vi "ograniczenie pwm6.vi"(10 "button 1":bool, 11 "X axis":i32) -> (3 "y":i16)   [LabVIEW 2015]
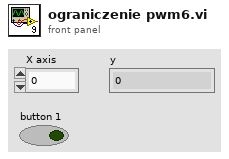
[diagram p1: front panel]
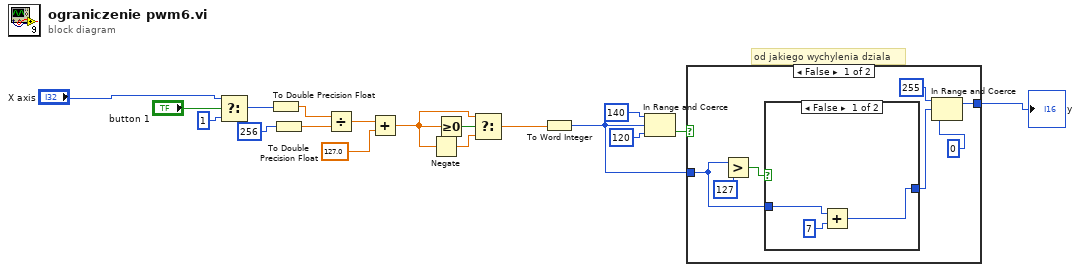
[diagram p0: block diagram]
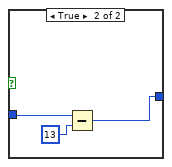
[diagram p2: hidden frame]
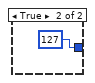
[diagram p3: hidden frame]
diagram:
  # "od jakiego wychylenia dziala"
  n1 = Select(t="X axis", s="button 1", f=1) -> (s? t:f=w1:i32)
  n2 = To Double Precision Float(number=w1) -> (double precision float=w2:dbl)
  n3 = To Double Precision Float(number=256 ("x")) -> (double precision float=w6:dbl)
  n4 = Divide(x=w2, y=w6) -> (x/y=w13:dbl)
  n5 = Add(x=w13, y=127.0 ("x")) -> (x+y=w12:dbl)
  n6 = Negate(x=w12) -> (-x=w14:dbl)
  n7 = Greater Or Equal To 0?(x=w12) -> (x >= 0?=w15:bool)
  n8 = Select(t=w12, s=w15, f=w14) -> (s? t:f=w10:dbl)
  n9 = To Word Integer(number=w10) -> (16bit integer=w9:i16)
  n10 = In Range and Coerce(upper limit=i16 140 ("y"), x=w9, lower limit=i16 120 ("y")) -> (In Range?=w16:bool)  [unwired: 1 out]
  n11 = case shown="False" w16 {
    tunnel: w9 -> [w20 _]
    tunnel: [w24 i16 127 ("y")] -> w8
    frame False {
      n12 = Greater?(x=w20, y=i16 127) -> (0:w21:bool)
      n13 = case shown="False" w21 {
        tunnel: [w26 w29] -> w23
        tunnel: w20 -> [w28 w31]
        frame False {
          n14 = Add(x=w28, y=i16 7) -> (x+y=w26:i16)
        }
        frame True {
          n15 = Subtract(x=w31, y=i16 13) -> (x-y=w29:i16)
        }
      }
      n16 = In Range and Coerce(upper limit=i16 255 ("y"), x=w23, lower limit=i16 0 ("y")) -> (coerced(x)=w24:i16)  [unwired: 1 out]
    }
    frame True {
    }
  }
  "y" <- w8
